vi "get file handle.vi"(8 "error in (no error)":errorcluster, 11 "Cascade in":refnum<class "Cascade.lvclass">) -> (0 "error out":errorcluster, 3 "Cascade out":refnum<class "Cascade.lvclass">)   [LabVIEW 2012, in "Cascade.lvclass"]
uses:
  Cascade.lvclass
  Cascade.lvclass/Cascade.ctl
panel:
  in  "FileName":string
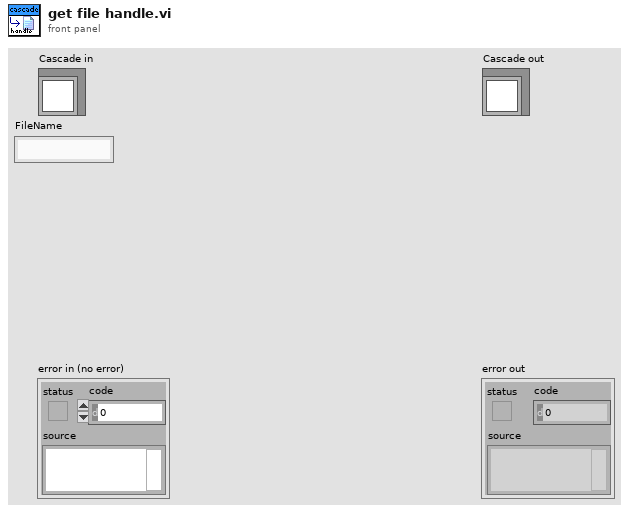
[diagram p1: front panel]
types:
  T1 = typedef "Cascade.lvclass/File type.ctl" = i32
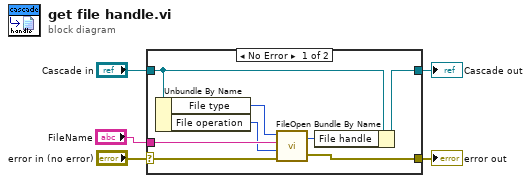
[diagram p0: block diagram]
diagram:
  n1 = case shown="No Error" "error in (no error)" {
    selector: "error in (no error)" -> [w13 w15]
    tunnel: [w12 w15] -> w4
    tunnel: [w7 w14] -> w2
    tunnel: "Cascade in" -> [w8 w14]
    tunnel: "FileName" -> [w10 _]
    frame No Error {
      n2 = Unbundle By Name(w8) -> ("File type"=w11:T1, "File operation"=w9:i32)
      n3 = call <userlib>:"FileOpen.vi"("error in"=w13, "File Operations"=w9, "FileName"=w10, "File Type"=w11) -> ("error out"=w12:errorcluster, "File Handle"=w6:u32)
      n4 = Bundle By Name(cluster=w8, "File handle"=w6) -> (w7:refnum<class "Cascade.lvclass">)
    }
    frame Error {
    }
  }
  "error out" <- w4
  "Cascade out" <- w2
